vi "GenerateFlow.vi"(0 "object in":refnum<class "CetoniPump.lvclass">, 1 "index":i32, 2 "Flow Rate":dbl, 5 "error in (no error)":errorcluster) -> (14 "object out":refnum<class "CetoniPump.lvclass">, 19 "error out":errorcluster)   [LabVIEW 2021, in "CetoniPump.lvclass"]
uses:
  CetoniPump.lvclass
  CetoniPump.lvclass/CetoniPump.ctl
  CETONI_SDK/lib/labview/labbCAN_Pump_API/labbCAN_Pump_API.lvlib
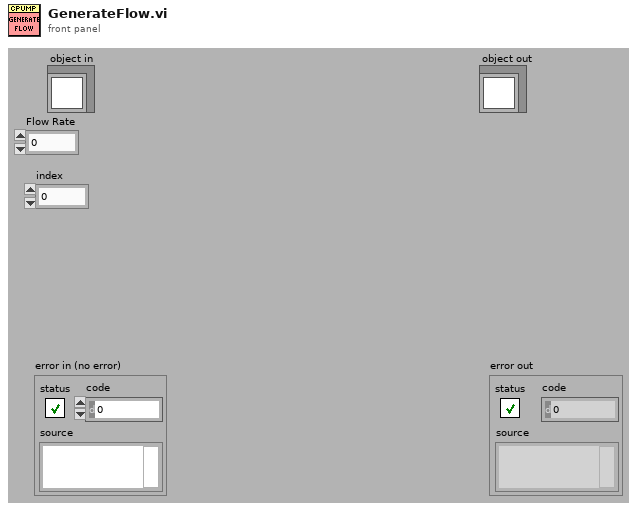
[diagram p1: front panel]
types:
  T1 = cluster{"Pump Handle":i64, "Pump Name":string, "Maximum Volume":dbl, "Maximum Flow Rate":dbl, "Flow Rate":dbl, "Target Level":dbl, "Valve Handle":i64, "Has Valve?":bool, "Actual valve position":i32}[]
  T2 = cluster{"Pump Handle":i64, "Pump Name":string, "Maximum Volume":dbl, "Maximum Flow Rate":dbl, "Flow Rate":dbl, "Target Level":dbl, "Valve Handle":i64, "Has Valve?":bool, "Actual valve position":i32}
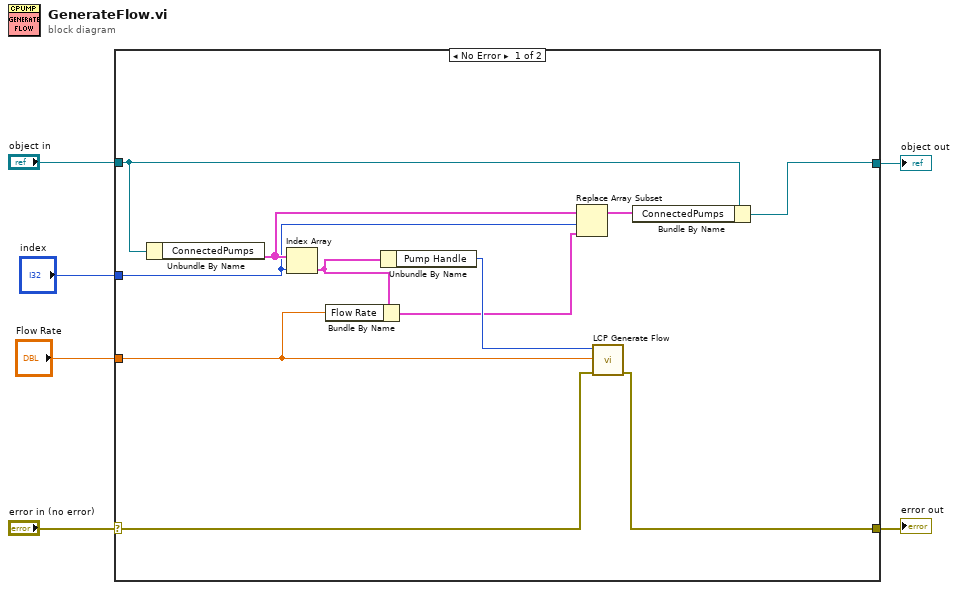
[diagram p0: block diagram]
diagram:
  n1 = case shown="No Error" "error in (no error)" {
    selector: "error in (no error)" -> [w17 w19]
    tunnel: [w16 w19] -> w5
    tunnel: [w8 w18] -> w3
    tunnel: "object in" -> [w7 w18]
    tunnel: "Flow Rate" -> [w11 _]
    tunnel: "index" -> [w13 _]
    frame No Error {
      n2 = Unbundle By Name(w7) -> ("ConnectedPumps"=w14:T1)
      n3 = Index Array(array=w14, index=w13) -> (element=w12:T2)
      n4 = Bundle By Name(cluster=w12, "Flow Rate"=w11) -> (w10:T2)
      n5 = Unbundle By Name(w12) -> ("Pump Handle"=w15:i64)
      n6 = Replace Array Subset(array=w14, new element=w10, index=w13) -> (w9:T1)
      n7 = call "LCP Generate Flow.vi"("error in (no error)"=w17, "Flow Rate"=w11, "Pump Handle"=w15) -> ("error out"=w16:errorcluster)  [unwired: 8 in]
      n8 = Bundle By Name(cluster=w7, "ConnectedPumps"=w9) -> (w8:refnum<class "CetoniPump.lvclass">)
    }
    frame Error {
    }
  }
  "error out" <- w5
  "object out" <- w3
